vi "Open File.vi"(8 "error in":errorcluster, 11 "CSV in":refnum<class "CSV.lvclass">) -> (0 "error out":errorcluster, 3 "CSV out":refnum<class "CSV.lvclass">)   [LabVIEW 2017, in "Report_lib.lvlib" / "CSV.lvclass"]
doc: "This method Open existing file with\npredefined FilePath for Read/Write"
uses:
  CSV.lvclass
  CSV.lvclass/CSV.ctl
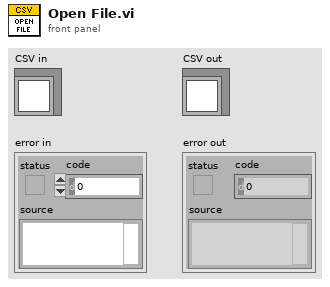
[diagram p1: front panel]
types:
  T1 = enum16{"open", "replace", "create", "open or create", "replace or create", "replace or create with confirmation"}
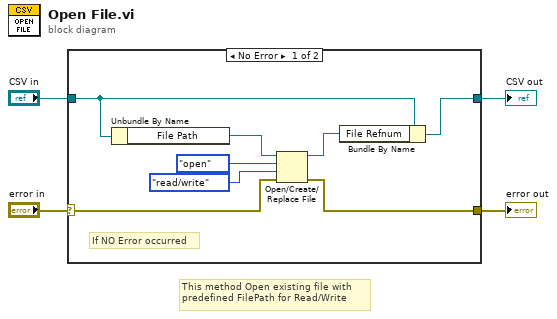
[diagram p0: block diagram]
diagram:
  # "This method Open existing file with\npredefined FilePath for Read/Write"
  n1 = case shown="No Error" "error in" {
    selector: "error in" -> [w6 w14]
    tunnel: [w5 w14] -> w3
    tunnel: [w7 w13] -> w1
    tunnel: "CSV in" -> [w8 w13]
    frame No Error {
      # "If NO Error occurred"
      n2 = Unbundle By Name(w8) -> ("File Path"=w10:path)
      n3 = Open/Create/Replace File(file path (use dialog)=w10, error in=w6, operation (0:open)=T1."open", access (0:read/write)=enum16{"read/write", "read-only", "write-only"}."read/write") -> (refnum out=w9:refnum<file>, error out=w5:errorcluster)  [unwired: 2 in, 1 out]
      n4 = Bundle By Name(cluster=w8, "File Refnum"=w9) -> (w7:refnum<class "CSV.lvclass">)
    }
    frame Error {
    }
  }
  "error out" <- w3
  "CSV out" <- w1
